vi "MGI Handle Menu.vi"(4 "SubObj":refnum<vi>, 5 "Control Enum":T2, 6 "Coord":T1, 7 "Activation? (F:Selection)":bool, 8 "error in (no error)":errorcluster, 9 "Activation:MenuRef":refnum<k9>, 10 "Selection:Menu Tag":string, 11 "MGI Error Reporter Dialog":refnum<class "MGI Error Reporter Dialog.lvclass">) -> (0 "error out":errorcluster, 1 "Activation:Discard?":bool, 3 "MGI Error Reporter Dialog Out":refnum<class "MGI Error Reporter Dialog.lvclass">)   [LabVIEW 2016, in "MGI Error Reporter Dialog.lvclass"]
doc: "Handle a Menu Activation Event or Menu Event in the Error Handler Dialog. This method defaults to allowing \"Explore\" option on the error path and \"Clear Error\", \"Clear All Errors\", and \"Export to Clipboard\" on the Error History listbox.\n\nAuthored by Shawn Walpole\nsupport@mooregoodideas.com\nwww.mooregoodideas.com\n\nCopyright (c) 2013, Moore Good Ideas, Inc.\n\nAll rights reserved.\n\nRedistribution and use in source and binary forms, with or without modification, are permitted provided that the following conditions are met:\n\n * Redistributions of source code must retain the above copyright notice, this list of conditions and the following disclaimer.\n * Redistributions in binary form must reproduce the above copyright notice, this list of conditions and the following disclaimer in the documentation and/or other materials provided with the distribution.\n * Neither the name of Moore Good Ideas, Inc. nor the names of its contributors may be used to endorse or promote products derived from this software without specific prior written permission.\n\nTHIS SOFTWARE IS PROVIDED BY THE COPYRIGHT HOLDERS AND CONTRIBUTORS \"AS IS\" AND ANY EXPRESS OR IMPLIED WARRANTIES, INCLUDING, BUT NOT LIMITED TO, THE IMPLIED WARRANTIES OF MERCHANTABILITY AND FITNESS FOR A PARTICULAR PURPOSE ARE DISCLAIMED. IN NO EVENT SHALL THE COPYRIGHT OWNER OR CONTRIBUTORS BE LIABLE FOR ANY DIRECT, INDIRECT, INCIDENTAL, SPECIAL, EXEMPLARY, OR CONSEQUENTIAL DAMAGES (INCLUDING, BUT NOT LIMITED TO, PROCUREMENT OF SUBSTITUTE GOODS OR SERVICES; LOSS OF USE, DATA, OR PROFITS; OR BUSINESS INTERRUPTION) HOWEVER CAUSED AND ON ANY THEORY OF LIABILITY, WHETHER IN CONTRACT, STRICT LIABILITY, OR TORT (INCLUDING NEGLIGENCE OR OTHERWISE) ARISING IN ANY WAY OUT OF THE USE OF THIS SOFTWARE, EVEN IF ADVISED OF THE POSSIBILITY OF SUCH DAMAGE."
uses:
  <userlib>/_MGI/Error Reporter/MGI Error Reporter Dialog/MGI Error Reporter Dialog.lvclass
  <userlib>/_MGI/Error Reporter/MGI Error Reporter Dialog/Protected/MGI Control Enum.ctl
  <vilib>/Utility/miscctls.llb/LVPoint32TypeDef.ctl
  C:/Program Files (x86)/National Instruments/LabVIEW 2016/user.lib/_MGI/Error Reporter/MGI Error Reporter Base/MGI Error Reporter Base.lvclass
  <userlib>/_MGI/Error Reporter/MGI Error Reporter Dialog/MGI Error Reporter Dialog.lvclass/MGI Error Reporter Dialog.ctl
  <userlib>/_MGI/Error Reporter/MGI Error Reporter Base/MGI Error Reporter Base.lvclass
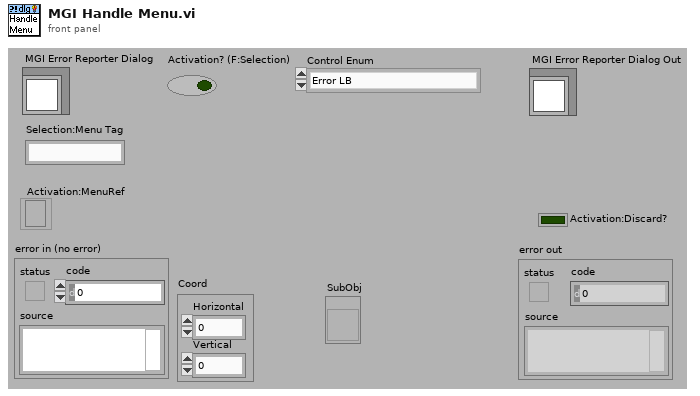
[diagram p1: front panel]
types:
  T1 = typedef "LVPoint32TypeDef.ctl" = cluster{"Horizontal":i32, "Vertical":i32}
  T2 = typedef "MGI Error Reporter Dialog.lvclass/MGI Control Enum.ctl" = enum16{"Error LB", "Details String", "Caller Ring", "Message String", "Clear Button"}
  T3 = typedef "MGI Error Reporter Dialog.lvclass/MGI Dialog UI Refs Cluster.ctl" = cluster{"LB Ref":refnum<vi>, "Details Ref":refnum<vi>, "Caller Ring Ref":refnum<vi>, "Message Ref":refnum<vi>, "Clear Btn Ref":refnum<vi>}
  T4 = typedef "LVRowAndColumnTypeDef.ctl" = cluster{"Row":i32, "Column":i32}
  T5 = enum32{"Invalid", "Default", "Floating", "Floating/Auto-Hide", "Modal"}
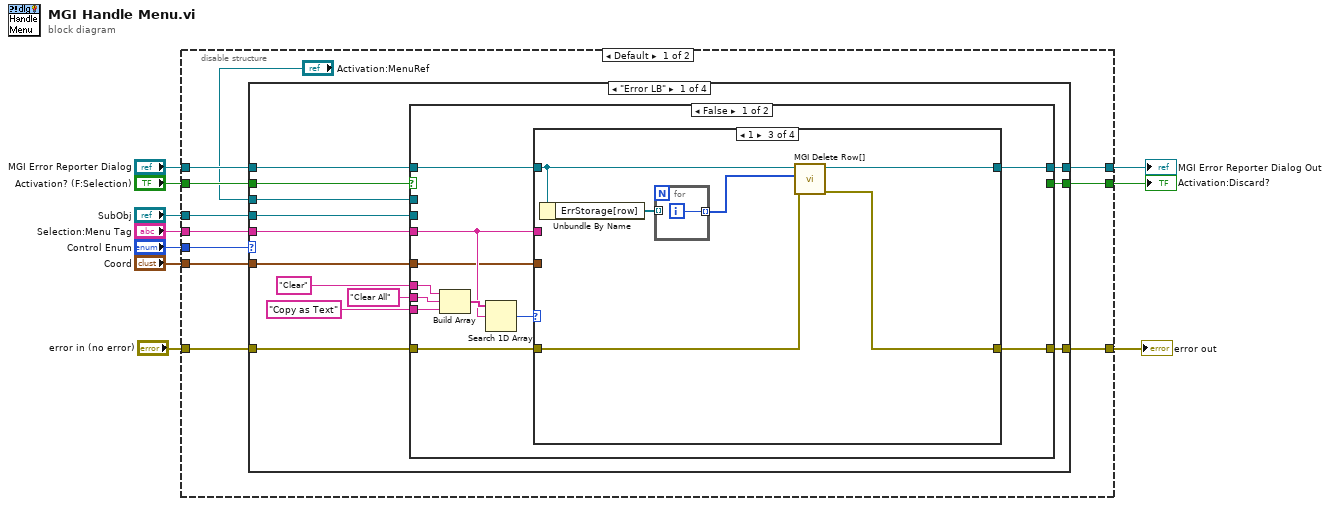
[diagram p0: block diagram]
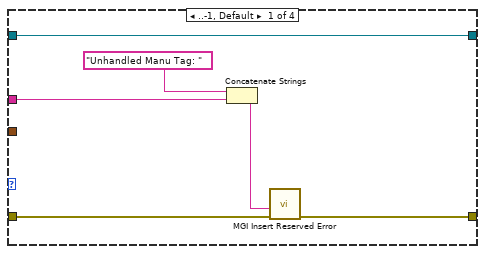
[diagram p2: hidden frame]
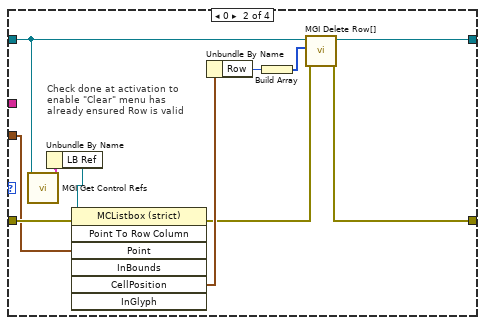
[diagram p3: hidden frame]
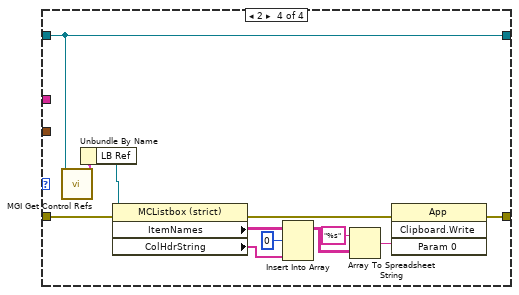
[diagram p4: hidden frame]
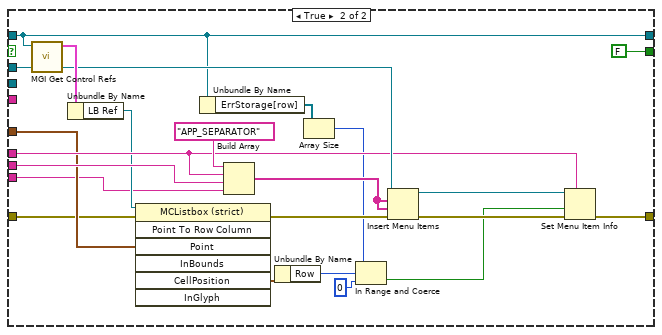
[diagram p5: hidden frame]
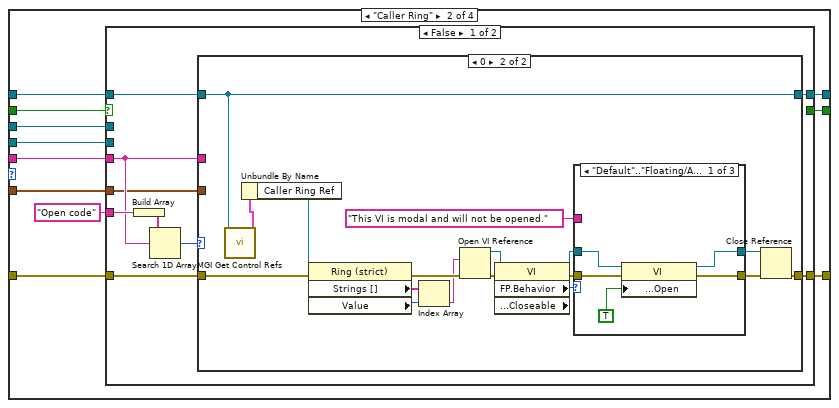
[diagram p6: hidden frame]
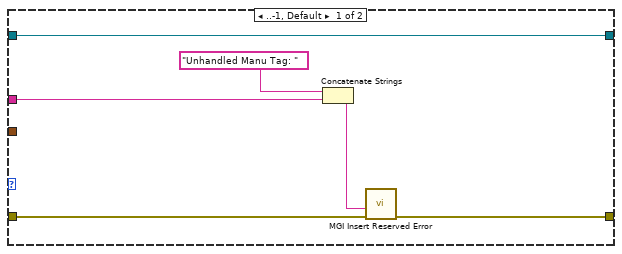
[diagram p7: hidden frame]
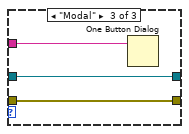
[diagram p9: hidden frame]
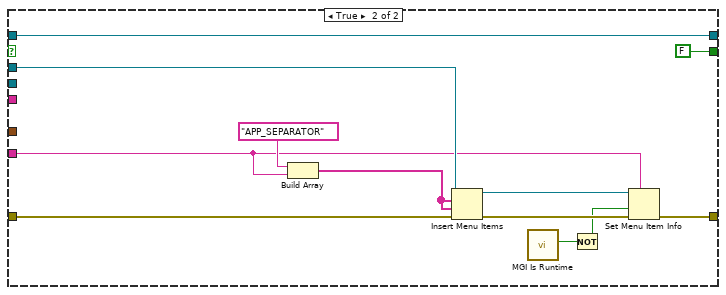
[diagram p10: hidden frame]
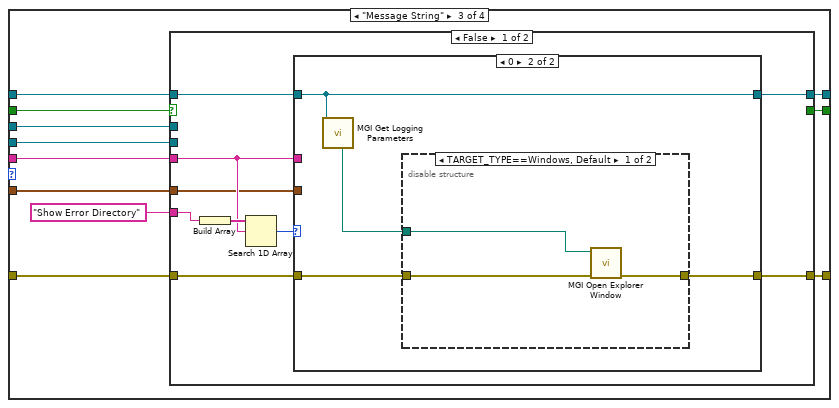
[diagram p11: hidden frame]
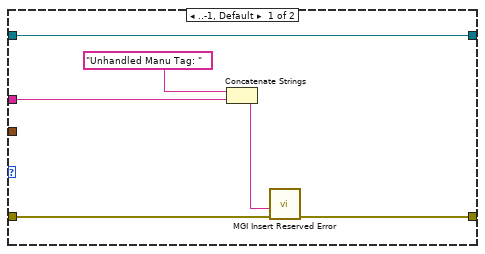
[diagram p12: hidden frame]
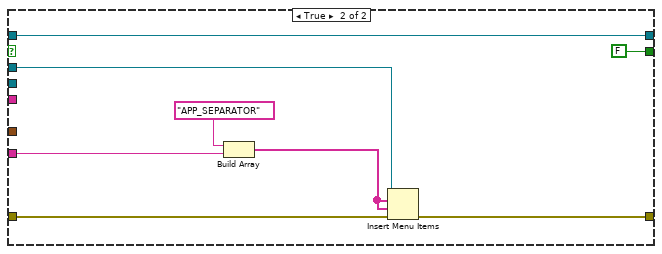
[diagram p14: hidden frame]
diagram:
  n1 = disable-structure shown="Default" {
    disable-tunnel: "Control Enum" -> [w21 _]
    disable-tunnel: "Activation? (F:Selection)" -> [w20 _]
    disable-tunnel: "SubObj" -> [w19 _]
    disable-tunnel: "Selection:Menu Tag" -> [w18 _]
    disable-tunnel: "Coord" -> [w17 _]
    disable-tunnel: [w16 _] -> w5
    disable-tunnel: "error in (no error)" -> [w15 w213]
    disable-tunnel: [w14 w213] -> w3
    disable-tunnel: "MGI Error Reporter Dialog" -> [w13 w214]
    disable-tunnel: [w12 w214] -> w1
    frame condition #0 (active) {
      n2 = case shown="\"Error LB\"" w21 {
        tunnel: w13 -> [w33 w113 w178 w212]
        tunnel: w20 -> [w34 w114 w179 _]
        tunnel: "Activation:MenuRef" -> [w32 w112 w177 _]
        tunnel: w19 -> [w31 w111 w176 _]
        tunnel: w18 -> [w30 w110 w175 _]
        tunnel: w17 -> [w29 w109 w174 _]
        tunnel: [w28 w108 w173 w212] -> w12
        tunnel: [w27 w107 w172 _] -> w16
        tunnel: w15 -> [w26 w106 w171 w211]
        tunnel: [w25 w105 w170 w211] -> w14
        frame "Error LB" {
          n3 = case shown="False" w34 {
            tunnel: w33 -> [w45 w85]
            tunnel: w32 -> [_ w101]
            tunnel: w31 -> [_ _]
            tunnel: w30 -> [w37 _]
            tunnel: w29 -> [w36 w92]
            tunnel: [w44 w85] -> w28
            tunnel: [_ FALSE] -> w27
            tunnel: w26 -> [w39 w91]
            tunnel: [w38 w96] -> w25
            tunnel: "Clear" -> [w43 w97]
            tunnel: "Clear All" -> [w42 w95]
            tunnel: "Copy as Text" -> [w35 w88]
            frame False {
              n4 = Build Array(w43, w42, w35) -> (w41:string[])
              n5 = Search 1D Array(1D array=w41, element=w37) -> (index of element=w40:i32)  [unwired: 1 out]
              n6 = case shown="1" w40 {
                tunnel: w45 -> [w51 w60 w65 w73]
                tunnel: [w51 w62 w68 w73] -> w44
                tunnel: w39 -> [w50 w57 w67 w79]
                tunnel: [w49 w61 w66 w74] -> w38
                tunnel: w37 -> [w48 _ _ _]
                tunnel: w36 -> [_ w56 _ _]
                frame ..-1, Default {
                  n7 = Concatenate Strings("Unhandled Manu Tag: " ("string"), w48) -> (w47:string)
                  n8 = call <userlib>:"MGI Insert Reserved Error.vi"("Error In"=w50, "Error Description"=w47) -> ("Error Out"=w49:errorcluster)  [unwired: 1 in, 8 out]
                }
                frame 0 {
                  # "Check done at activation to enable \"Clear\" menu has already ensured Row is valid"
                  n9 = call <userlib>:"MGI Get Control Refs.vi"("MGI Error Dialog.lvclass"=w60) -> ("Refs"=w59:T3)  [unwired: 10 out]
                  n10 = Unbundle By Name(w59) -> ("LB Ref"=w58:refnum<vi>)
                  n11 = invoke class="MCListbox (strict)" method="Point To Row Column"(reference=w58, error in=w57, "Point"=w56) -> (error out=w54:errorcluster, "CellPosition"=w55:T4)  [unwired: 4 in, 5 out]
                  n12 = Unbundle By Name(w55) -> ("Row"=w53:i32)
                  n13 = Build Array(w53) -> (w52:i32[])
                  n14 = call-dynamic "MGI Delete Row[].vi"("error in (no error)"=w54, "Listbox row[] to delete"=w52, "MGI Error Handler in"=w60) -> ("error out"=w61:errorcluster, "MGI Error Handler out"=w62:refnum<class "MGI Error Reporter Dialog.lvclass">)  [unwired: 7 out]
                }
                frame 1 {
                  n15 = Unbundle By Name(w65) -> ("ErrStorage[row]"=w64:refnum<class "MGI ERD LB Row Base.lvclass">[])
                  n16 = for {
                    tunnel: w64 -> [_] mode=indexing
                    tunnel: [w69] -> w63 mode=indexing
                    i -> [w69]
                  }
                  n17 = call-dynamic "MGI Delete Row[].vi"("error in (no error)"=w67, "Listbox row[] to delete"=w63, "MGI Error Handler in"=w65) -> ("error out"=w66:errorcluster, "MGI Error Handler out"=w68:refnum<class "MGI Error Reporter Dialog.lvclass">)  [unwired: 7 out]
                }
                frame 2 {
                  n18 = call <userlib>:"MGI Get Control Refs.vi"("MGI Error Dialog.lvclass"=w73) -> ("Refs"=w81:T3)  [unwired: 10 out]
                  n19 = Unbundle By Name(w81) -> ("LB Ref"=w80:refnum<vi>)
                  n20 = property class="MCListbox (strict)"(reference=w80, error in=w79) -> (error out=w75:errorcluster, "ItemNames"=w78:string[][], "ColHdrString"=w77:string[])  [unwired: 1 out]
                  n21 = Insert Into Array(array=w78, index (row)=0, new element=w77) -> (w72:string[][])  [unwired: 1 in]
                  n22 = Array To Spreadsheet String(array=w72, 3:"%s" ("format string")) -> (spreadsheet string=w71:string)  [unwired: 1 out]
                  n23 = invoke class="App" method="Clipboard.Write"(error in=w75, "Param 0"=w71) -> (error out=w74:errorcluster)  [unwired: 2 in, 3 out]
                }
              }
            }
            frame True {
              n24 = call <userlib>:"MGI Get Control Refs.vi"("MGI Error Dialog.lvclass"=w85) -> ("Refs"=w102:T3)  [unwired: 10 out]
              n25 = Unbundle By Name(w102) -> ("LB Ref"=w93:refnum<vi>)
              n26 = invoke class="MCListbox (strict)" method="Point To Row Column"(reference=w93, error in=w91, "Point"=w92) -> (error out=w90:errorcluster, "CellPosition"=w89:T4)  [unwired: 4 in, 5 out]
              n27 = Unbundle By Name(w85) -> ("ErrStorage[row]"=w84:refnum<class "MGI ERD LB Row Base.lvclass">[])
              n28 = Build Array("APP_SEPARATOR", w97, w95, w88) -> (w94:string[])
              n29 = Unbundle By Name(w89) -> ("Row"=w87:i32)
              n30 = Array Size(array=w84) -> (size(s)=w83:i32)
              n31 = In Range and Coerce(upper limit=w83, x=w87, lower limit=0) -> (In Range?=w82:bool)  [unwired: 1 out]
              n32 = Insert Menu Items(6:w90, 7:w94, 8:w94, 9:w101) -> (0:w100:errorcluster, 3:w99:refnum<k9>)  [unwired: 3 out]
              n33 = Set Menu Item Info(7:w97, 8:w100, 9:w82, 11:w99) -> (0:w96:errorcluster)  [unwired: 4 out]
            }
          }
        }
        frame "Caller Ring" {
          n34 = case shown="False" w114 {
            tunnel: w113 -> [w123 w160]
            tunnel: w112 -> [_ w167]
            tunnel: w111 -> [_ _]
            tunnel: w110 -> [w116 _]
            tunnel: w109 -> [w115 _]
            tunnel: [w122 w160] -> w108
            tunnel: [_ FALSE] -> w107
            tunnel: w106 -> [w118 w159]
            tunnel: [w117 w162] -> w105
            tunnel: "Open code" -> [w121 w163]
            frame False {
              n35 = Build Array(w121) -> (w120:string[])
              n36 = Search 1D Array(1D array=w120, element=w116) -> (index of element=w119:i32)  [unwired: 1 out]
              n37 = case shown="0" w119 {
                tunnel: w123 -> [w129 w143]
                tunnel: [w129 w143] -> w122
                tunnel: w118 -> [w128 w144]
                tunnel: [w127 w134] -> w117
                tunnel: w116 -> [w126 _]
                tunnel: w115 -> [_ _]
                frame ..-1, Default {
                  n38 = Concatenate Strings("Unhandled Manu Tag: " ("string"), w126) -> (w125:string)
                  n39 = call <userlib>:"MGI Insert Reserved Error.vi"("Error In"=w128, "Error Description"=w125) -> ("Error Out"=w127:errorcluster)  [unwired: 1 in, 8 out]
                }
                frame 0 {
                  n40 = call <userlib>:"MGI Get Control Refs.vi"("MGI Error Dialog.lvclass"=w143) -> ("Refs"=w146:T3)  [unwired: 10 out]
                  n41 = Unbundle By Name(w146) -> ("Caller Ring Ref"=w145:refnum<vi>)
                  n42 = property class="Ring (strict)"(reference=w145, error in=w144) -> (error out=w133:errorcluster, "Strings []"=w132:string[], "Value"=w131:u16)  [unwired: 1 out]
                  n43 = Index Array(array=w132, index=w131) -> (element=w130:string)
                  n44 = Open VI Reference(vi path=w130, error in (no error)=w133) -> (vi reference=w135:refnum<vi>, error out=w136:errorcluster)  [unwired: 4 out]
                  n45 = property class="VI" props=["FP.Behavior", "Front Panel.Closeable"](reference=w135, error in=w136) -> (reference out=w140:refnum<vi>, error out=w138:errorcluster, "FP.Behavior"=w137:T5)  [unwired: 1 out]
                  n46 = case shown="\"Default\"..\"Floating/Auto-Hide\"" w137 {
                    tunnel: w138 -> [w148 w152 w156]
                    tunnel: [w149 w152 w156] -> w139
                    tunnel: w140 -> [w147 w153 w155]
                    tunnel: [w150 w153 w155] -> w141
                    tunnel: "This VI is modal and will not be opened." ("message") -> [_ _ w154]
                    frame "Default".."Floating/Auto-Hide" {
                      n47 = property class="VI"(reference=w147, error in=w148, "Block Diagram Window:Open"=TRUE ("Activate?")) -> (reference out=w150:refnum<vi>, error out=w149:errorcluster)
                    }
                    frame "Invalid", Default {
                    }
                    frame "Modal" {
                      n48 = One Button Dialog(message=w154) -> ()  [unwired: 2 out]
                    }
                  }
                  n49 = Close Reference(reference=w141, error in (no error)=w139) -> (error out=w134:errorcluster)
                }
              }
            }
            frame True {
              n50 = Build Array("APP_SEPARATOR", w163) -> (w161:string[])
              n51 = Insert Menu Items(6:w159, 7:w161, 8:w161, 9:w167) -> (0:w166:errorcluster, 3:w165:refnum<k9>)  [unwired: 3 out]
              n52 = call <userlib>:"MGI Is Runtime.vi"() -> ("Run Time System?"=w158:bool)  [unwired: 7 out]
              n53 = Not(x=w158) -> (.not. x?=w157:bool)
              n54 = Set Menu Item Info(7:w163, 8:w166, 9:w157, 11:w165) -> (0:w162:errorcluster)  [unwired: 4 out]
            }
          }
        }
        frame "Message String" {
          n55 = case shown="False" w179 {
            tunnel: w178 -> [w188 w205]
            tunnel: w177 -> [_ w209]
            tunnel: w176 -> [_ _]
            tunnel: w175 -> [w181 _]
            tunnel: w174 -> [w180 _]
            tunnel: [w187 w205] -> w173
            tunnel: [_ FALSE] -> w172
            tunnel: w171 -> [w183 w204]
            tunnel: [w182 w203] -> w170
            tunnel: "Show Error Directory" -> [w186 w207]
            frame False {
              n56 = Build Array(w186) -> (w185:string[])
              n57 = Search 1D Array(1D array=w185, element=w181) -> (index of element=w184:i32)  [unwired: 1 out]
              n58 = case shown="0" w184 {
                tunnel: w188 -> [w194 w197]
                tunnel: [w194 w197] -> w187
                tunnel: w183 -> [w193 w198]
                tunnel: [w192 w195] -> w182
                tunnel: w181 -> [w191 _]
                tunnel: w180 -> [_ _]
                frame ..-1, Default {
                  n59 = Concatenate Strings("Unhandled Manu Tag: " ("string"), w191) -> (w190:string)
                  n60 = call <userlib>:"MGI Insert Reserved Error.vi"("Error In"=w193, "Error Description"=w190) -> ("Error Out"=w192:errorcluster)  [unwired: 1 in, 8 out]
                }
                frame 0 {
                  n61 = call <userlib>:"MGI Get Logging Parameters.vi"("MGI Error Reporter Base"=w197) -> ("Error Log Directory"=w196:path)  [unwired: 10 out]
                  n62 = disable-structure shown="TARGET_TYPE==Windows, Default" {
                    disable-tunnel: w198 -> [w200 w202]
                    disable-tunnel: w196 -> [w199 _]
                    disable-tunnel: [w201 w202] -> w195
                    frame condition #0 (active) {
                      n63 = call <userlib>:"MGI Open Explorer Window.vi"("error in (no error)"=w200, "Directory or File"=w199) -> ("error out"=w201:errorcluster)  [unwired: 9 out]
                    }
                    frame condition #1 {
                    }
                  }
                }
              }
            }
            frame True {
              n64 = Build Array("APP_SEPARATOR", w207) -> (w206:string[])
              n65 = Insert Menu Items(6:w204, 7:w206, 8:w206, 9:w209) -> (0:w203:errorcluster)  [unwired: 4 out]
            }
          }
        }
        frame "Details String", "Clear Button" {
        }
      }
    }
    frame condition #1 {
    }
  }
  "Activation:Discard?" <- w5
  "error out" <- w3
  "MGI Error Reporter Dialog Out" <- w1
